vi "Lettura 3 Proximity_fin.vi"() -> ()   [LabVIEW 2020]
uses:
  <vilib>/DAQmx/read.llb/DAQmx Read (Analog 1D Wfm NChan NSamp).vi
  <vilib>/Analysis/baseanly.llb/Mean (DBL).vi
  <vilib>/DAQmx/configure/timing.llb/DAQmx Timing (Sample Clock).vi
  <vilib>/DAQmx/miscellaneous.llb/DAQmx Fill In Error Info.vi
  <vilib>/Utility/file.llb/Write Delimited Spreadsheet (DBL).vi
  <vilib>/Analysis/NI_AALBase.lvlib
panel:
  in  "File txt Tensione 1":path
  out "Distanza 1":dbl[](graph)
  in  "File txt Distanza 1":path
  out "Media 3":dbl format="%0.2f"
  out "Deviazione Standard 3":dbl format="%0.2f"
  out "Massimo3":dbl
  out "Minimo 3":dbl
  in  "File txt Tensione 2":path
  out "Distanza 2":dbl[](graph)
  in  "File txt Distanza 2":path
  out "Media 2":dbl format="%0.2f"
  out "Deviazione Standard 2":dbl format="%0.2f"
  out "Massimo 2":dbl
  out "Minimo 2":dbl
  out "Segnale Proximity 1":dynamicdata(graph)
  out "Segnale Proximity 2":dynamicdata(graph)
  out "Minimo":dbl
  out "Massimo":dbl
  out "Deviazione Standard":dbl format="%0.2f"
  out "Media":dbl format="%0.2f"
  in  "File txt Distanza 3":path
  out "Distanza 3":dbl[](graph)
  out "Segnale Proximity 3":dynamicdata(graph)
  out "num campioni":dbl
  in  "File txt Tensione 3":path
  in  "SAVE":bool
  in  "Frequenza":dbl=5000.0 format="%0.2p"
  in  "Durata":dbl=0.1 format="%.2p"
  in  "STOP":bool
  out "current time":timestamp
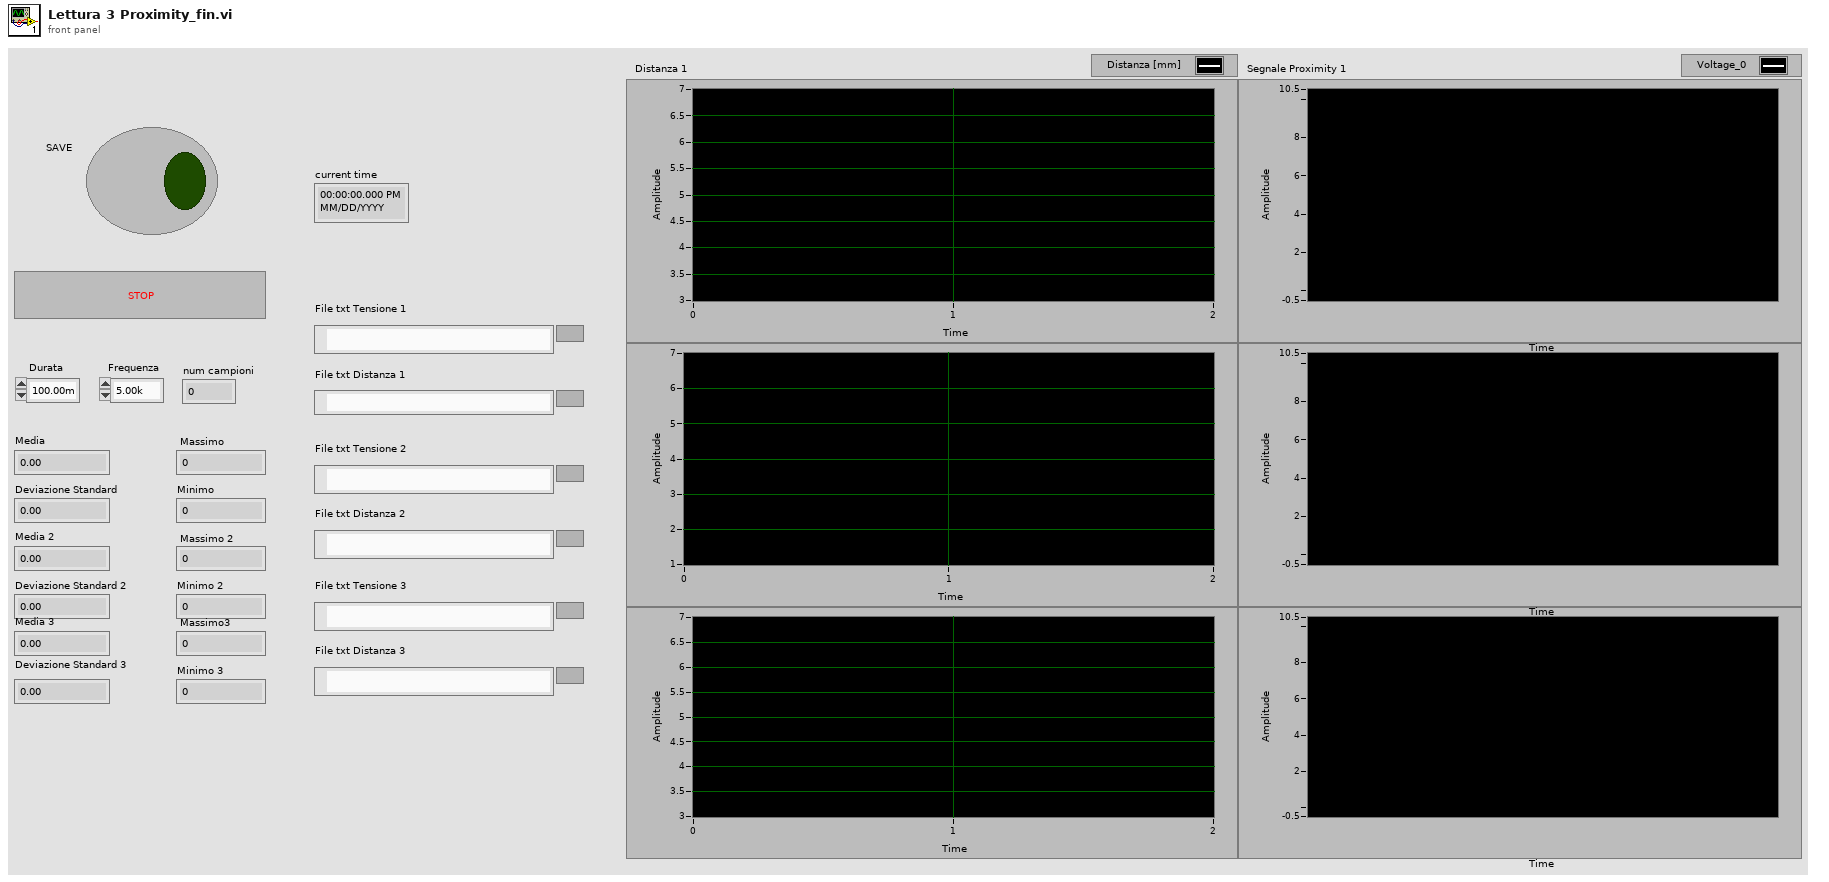
[diagram p1: front panel]
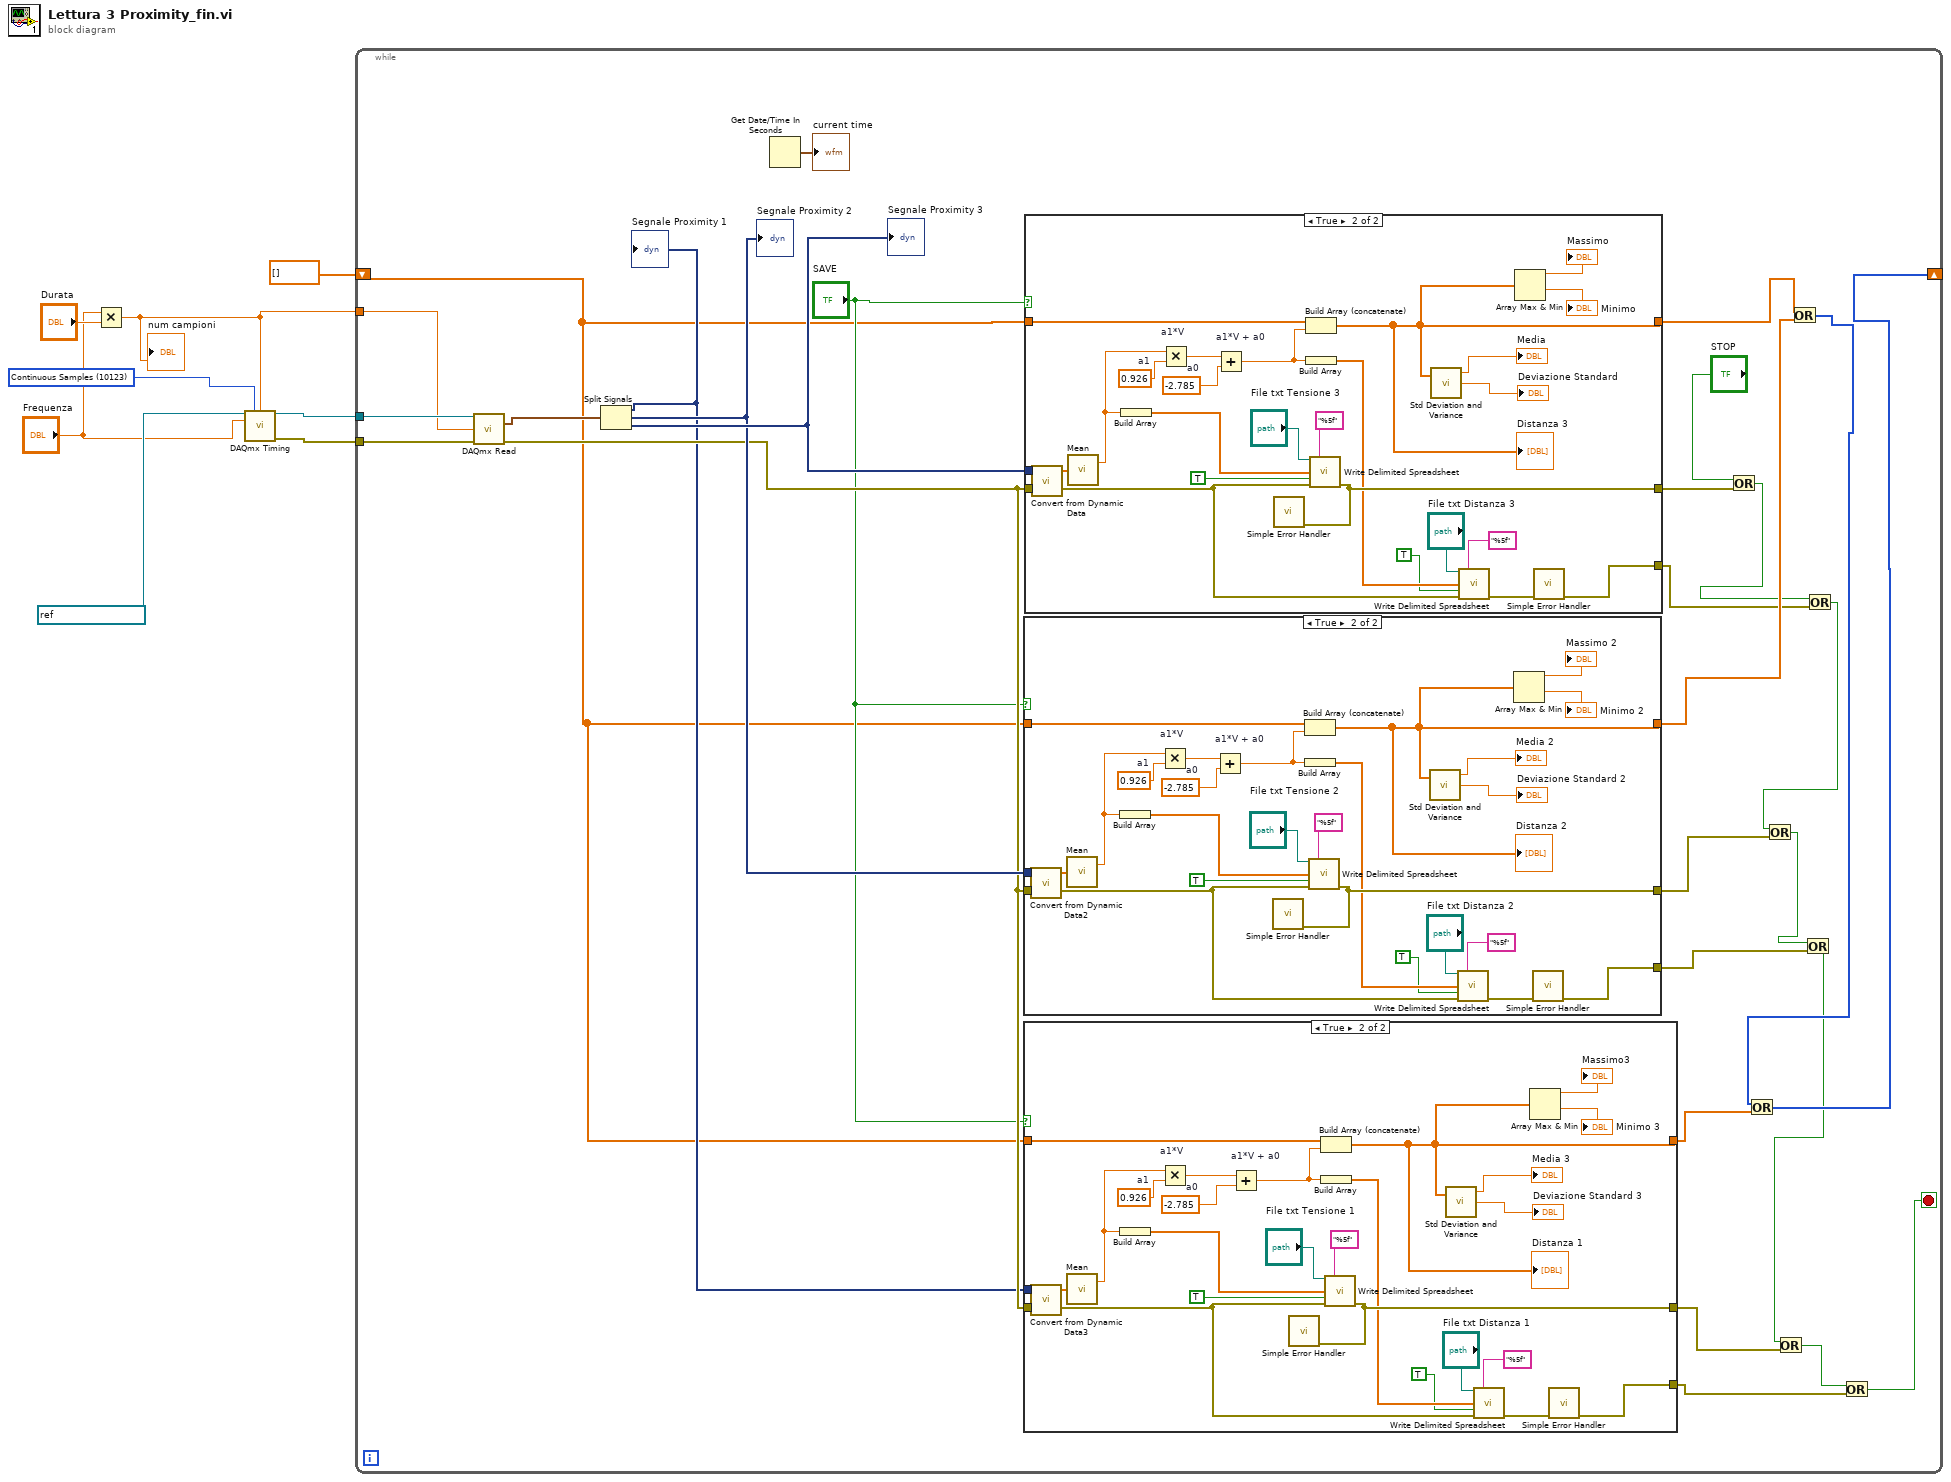
[diagram p0: block diagram]
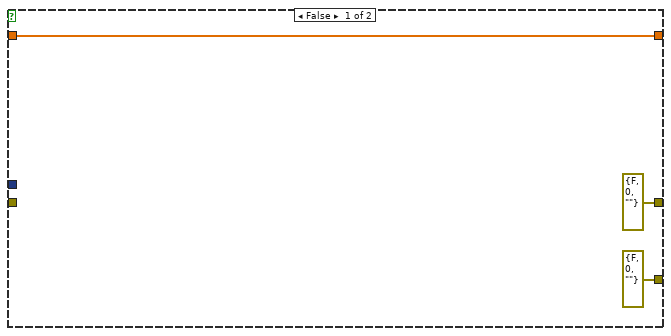
[diagram p2: hidden frame]
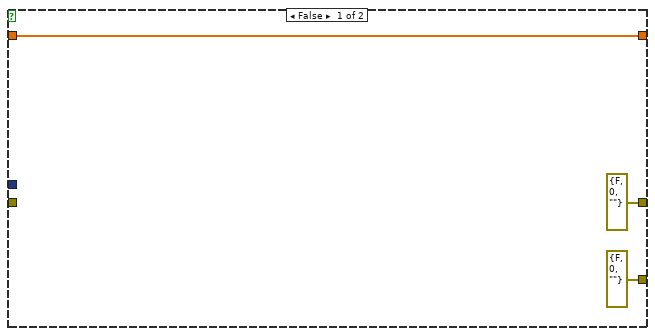
[diagram p3: hidden frame]
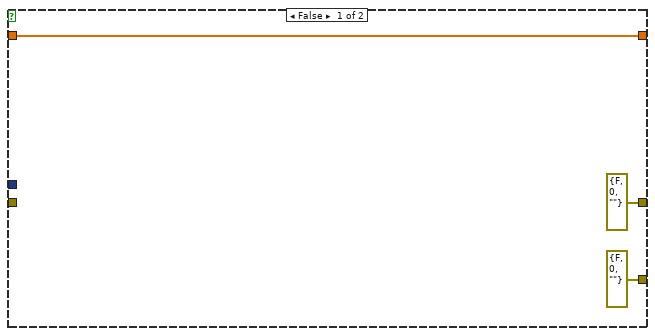
[diagram p4: hidden frame]
diagram:
  w4 = 10123 items=["Finite Samples"=10178, "Continuous Samples"=10123, "Hardware Timed Single Point"=12522] ("sample mode")
  n1 = Multiply(x="Frequenza", y="Durata") -> (x*y=w5:dbl)
  "num campioni" <- w5
  n2 = call-poly <vilib>:"DAQmx Timing.vi"("task/channels in"=refnum<k21> "MyVoltageTask", "sample mode"=w4, "samples per channel"=w5, "rate"="Frequenza") -> ("task out"=w8:refnum<k21>, "error out"=w3:errorcluster)  [unwired: 10 in]
  n3 = while {
    tunnel: w8 -> [w36]
    tunnel: w5 -> [w35]
    tunnel: w3 -> [w34]
    shift-right: [w21] -> _
    shift-left: dbl[] [] -> [w17]
    stop <- w9 stop-if-true
    n4 = call-poly <vilib>:"DAQmx Read.vi"("task/channels in"=w36, "number of samples per channel"=w35, "error in"=w34) -> ("data"=w32:waveform(dbl)[], "error out"=w20:errorcluster)  [unwired: 10 in, 1 out]
    n5 = Split Signals(w32) -> (w19:dynamicdata, w30:dynamicdata, w31:dynamicdata)  [unwired: 3 in]
    "Segnale Proximity 3" <- w31
    "Segnale Proximity 2" <- w30
    "Segnale Proximity 1" <- w19
    n6 = Get Date/Time In Seconds() -> (seconds since 1Jan1904=→"current time":timestamp)
    n7 = case shown="True" "SAVE" {
      tunnel: [errorcluster {"status"=FALSE, "code"=0, "source"=""} ("error IO") w92] -> w27
      tunnel: w30 -> [_ w91]
      tunnel: w20 -> [_ w84]
      tunnel: [w67 w72] -> w29
      tunnel: w17 -> [w67 w75]
      tunnel: [errorcluster {"status"=FALSE, "code"=0, "source"=""} ("error out") w82] -> w23
      frame False {
      }
      frame True {
        w77 = -2.785  # a0
        w78 = 0.926  # a1
        n8 = call "Convert from Dynamic Data2"("Dynamic Data Type"=w91) -> ("Array"=w69:dbl[])  [unwired: 3 in]
        n9 = call-poly <vilib>:"Mean.vi"("X"=w69) -> ("mean"=w79:dbl)  [unwired: 1 out]
        n10 = Build Array(w79) -> (w88:dbl[])
        n11 = Multiply "a1*V"(x=w79, y=w78) -> (x*y=w80:dbl)
        n12 = Add "a1*V + a0"(x=w80, y=w77) -> (x+y=w76:dbl)
        n13 = Build Array (concatenate)(w75, w76) -> (w72:dbl[])
        "Distanza 2" <- w72
        n14 = Build Array(w76) -> (w87:dbl[])
        n15 = call-poly <vilib>:"Write Delimited Spreadsheet.vi"("file path (dialog if empty)"="File txt Tensione 2", "format (%.3f)"="%5f", "1D data"=w88, "append to file? (new file:F)"=TRUE, "error in (no error)"=w84) -> ("error out"=w92:errorcluster)  [unwired: 9 in, 1 out]
        n16 = call <vilib>:"Simple Error Handler.vi"("error in (no error)"=w92) -> ()  [unwired: 4 in, 5 out]
        n17 = call <vilib>:"Std Deviation and Variance.vi"("X"=w72) -> ("mean"=→"Media 2":dbl, "standard deviation"=→"Deviazione Standard 2":dbl)  [unwired: 1 in, 1 out]
        n18 = call-poly <vilib>:"Write Delimited Spreadsheet.vi"("file path (dialog if empty)"="File txt Distanza 2", "format (%.3f)"="%5f", "1D data"=w87, "append to file? (new file:F)"=TRUE, "error in (no error)"=w84) -> ("error out"=w83:errorcluster)  [unwired: 9 in, 1 out]
        n19 = Array Max & Min(array=w72) -> (max value=→"Massimo 2":dbl, min value=→"Minimo 2":dbl)  [unwired: 2 out]
        n20 = call <vilib>:"Simple Error Handler.vi"("error in (no error)"=w83) -> ("error out"=w82:errorcluster)  [unwired: 4 in, 4 out]
      }
    }
    n21 = case shown="True" "SAVE" {
      tunnel: [errorcluster {"status"=FALSE, "code"=0, "source"=""} ("error IO") w64] -> w26
      tunnel: w19 -> [_ w63]
      tunnel: w20 -> [_ w56]
      tunnel: [w39 w44] -> w24
      tunnel: w17 -> [w39 w47]
      tunnel: [errorcluster {"status"=FALSE, "code"=0, "source"=""} ("error out") w54] -> w25
      frame False {
      }
      frame True {
        w49 = -2.785  # a0
        w50 = 0.926  # a1
        n22 = call "Convert from Dynamic Data3"("Dynamic Data Type"=w63) -> ("Array"=w41:dbl[])  [unwired: 3 in]
        n23 = call-poly <vilib>:"Mean.vi"("X"=w41) -> ("mean"=w51:dbl)  [unwired: 1 out]
        n24 = Build Array(w51) -> (w60:dbl[])
        n25 = Multiply "a1*V"(x=w51, y=w50) -> (x*y=w52:dbl)
        n26 = Add "a1*V + a0"(x=w52, y=w49) -> (x+y=w48:dbl)
        n27 = Build Array (concatenate)(w47, w48) -> (w44:dbl[])
        "Distanza 1" <- w44
        n28 = Build Array(w48) -> (w59:dbl[])
        n29 = call-poly <vilib>:"Write Delimited Spreadsheet.vi"("file path (dialog if empty)"="File txt Tensione 1", "format (%.3f)"="%5f", "1D data"=w60, "append to file? (new file:F)"=TRUE, "error in (no error)"=w56) -> ("error out"=w64:errorcluster)  [unwired: 9 in, 1 out]
        n30 = call <vilib>:"Simple Error Handler.vi"("error in (no error)"=w64) -> ()  [unwired: 4 in, 5 out]
        n31 = call <vilib>:"Std Deviation and Variance.vi"("X"=w44) -> ("mean"=→"Media 3":dbl, "standard deviation"=→"Deviazione Standard 3":dbl)  [unwired: 1 in, 1 out]
        n32 = call-poly <vilib>:"Write Delimited Spreadsheet.vi"("file path (dialog if empty)"="File txt Distanza 1", "format (%.3f)"="%5f", "1D data"=w59, "append to file? (new file:F)"=TRUE, "error in (no error)"=w56) -> ("error out"=w55:errorcluster)  [unwired: 9 in, 1 out]
        n33 = Array Max & Min(array=w44) -> (max value=→"Massimo3":dbl, min value=→"Minimo 3":dbl)  [unwired: 2 out]
        n34 = call <vilib>:"Simple Error Handler.vi"("error in (no error)"=w55) -> ("error out"=w54:errorcluster)  [unwired: 4 in, 4 out]
      }
    }
    n35 = case shown="True" "SAVE" {
      tunnel: [errorcluster {"status"=FALSE, "code"=0, "source"=""} ("error IO") w120] -> w13
      tunnel: w31 -> [_ w119]
      tunnel: w20 -> [_ w112]
      tunnel: [w95 w100] -> w28
      tunnel: w17 -> [w95 w103]
      tunnel: [errorcluster {"status"=FALSE, "code"=0, "source"=""} ("error out") w110] -> w15
      frame False {
      }
      frame True {
        w105 = -2.785  # a0
        w106 = 0.926  # a1
        n36 = call "Convert from Dynamic Data"("Dynamic Data Type"=w119) -> ("Array"=w97:dbl[])  [unwired: 3 in]
        n37 = call-poly <vilib>:"Mean.vi"("X"=w97) -> ("mean"=w107:dbl)  [unwired: 1 out]
        n38 = Build Array(w107) -> (w116:dbl[])
        n39 = Multiply "a1*V"(x=w107, y=w106) -> (x*y=w108:dbl)
        n40 = Add "a1*V + a0"(x=w108, y=w105) -> (x+y=w104:dbl)
        n41 = Build Array (concatenate)(w103, w104) -> (w100:dbl[])
        "Distanza 3" <- w100
        n42 = Build Array(w104) -> (w115:dbl[])
        n43 = call-poly <vilib>:"Write Delimited Spreadsheet.vi"("file path (dialog if empty)"="File txt Tensione 3", "format (%.3f)"="%5f", "1D data"=w116, "append to file? (new file:F)"=TRUE, "error in (no error)"=w112) -> ("error out"=w120:errorcluster)  [unwired: 9 in, 1 out]
        n44 = call <vilib>:"Simple Error Handler.vi"("error in (no error)"=w120) -> ()  [unwired: 4 in, 5 out]
        n45 = call <vilib>:"Std Deviation and Variance.vi"("X"=w100) -> ("mean"=→"Media":dbl, "standard deviation"=→"Deviazione Standard":dbl)  [unwired: 1 in, 1 out]
        n46 = call-poly <vilib>:"Write Delimited Spreadsheet.vi"("file path (dialog if empty)"="File txt Distanza 3", "format (%.3f)"="%5f", "1D data"=w115, "append to file? (new file:F)"=TRUE, "error in (no error)"=w112) -> ("error out"=w111:errorcluster)  [unwired: 9 in, 1 out]
        n47 = Array Max & Min(array=w100) -> (max value=→"Massimo":dbl, min value=→"Minimo":dbl)  [unwired: 2 out]
        n48 = call <vilib>:"Simple Error Handler.vi"("error in (no error)"=w111) -> ("error out"=w110:errorcluster)  [unwired: 4 in, 4 out]
      }
    }
    n49 = Or(x="STOP", y=w13) -> (x .or. y?=w14:bool)
    n50 = Or(x=w28, y=w29) -> (x .or. y?=w22:i32[])
    n51 = Or(x=w22, y=w24) -> (x .or. y?=w21:i32[])
    n52 = Or(x=w14, y=w15) -> (x .or. y?=w11:bool)
    n53 = Or(x=w11, y=w27) -> (x .or. y?=w10:bool)
    n54 = Or(x=w10, y=w23) -> (x .or. y?=w12:bool)
    n55 = Or(x=w12, y=w26) -> (x .or. y?=w16:bool)
    n56 = Or(x=w16, y=w25) -> (x .or. y?=w9:bool)
  }
